vi "Power Keep Sign.vi"(1 "Power":dbl, 2 "In":dbl) -> (0 "Out":dbl)   [LabVIEW 2013]
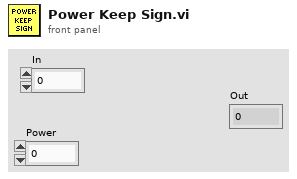
[diagram p1: front panel]
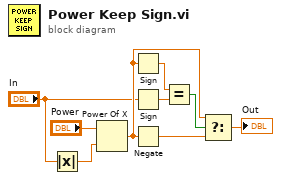
[diagram p0: block diagram]
diagram:
  n1 = Absolute Value(x="In") -> (abs(x)=w2:dbl)
  n2 = Power Of X(1:w2, 2:"Power") -> (0:w3:dbl)
  n3 = Sign(1:w3) -> (0:w7:dbl)
  n4 = Sign(1:"In") -> (0:w8:dbl)
  n5 = Negate(x=w3) -> (-x=w4:dbl)
  n6 = Equal?(x=w7, y=w8) -> (x = y?=w6:bool)
  n7 = Select(t=w3, s=w6, f=w4) -> (s? t:f=→"Out":dbl)
